vi "ReadObjectLayout.vi"(7 "properties to ignore":variant, 8 "error in (no error)":errorcluster, 10 "GObj Refnum":refnum<vi>, 11 "Control Layout in":refnum<class "Control Layout.lvclass">) -> (0 "error out":errorcluster, 3 "Control Layout out":refnum<class "Control Layout.lvclass">)   [LabVIEW 2010, in "NI_SE_Front Panel Layout.lvlib" / "Control Layout.lvclass"]
doc: "Read layout information from the GObj Refnum."
uses:
  Control Layout.lvclass
  Object Layout/Object Layout.lvclass
  Control Layout.lvclass/Control Layout.ctl
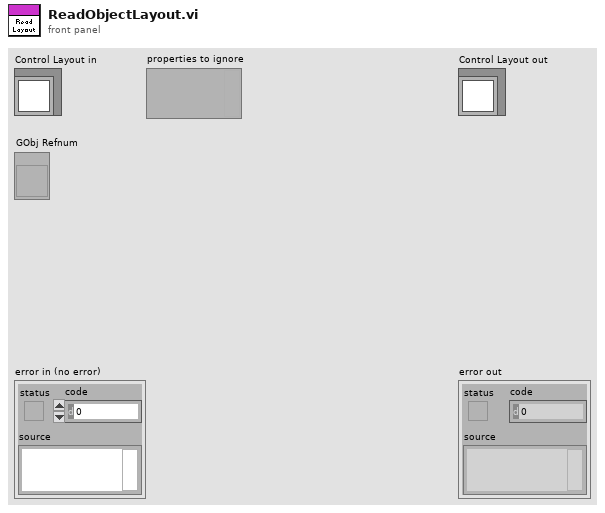
[diagram p1: front panel]
types:
  T1 = typedef "LVFontTypeDef.ctl" = cluster{"Font Name":string, "Size":u16, "Bold":bool, "Italic":bool, "Underline":bool, "Strikeout":bool, "Color":u32}
  T2 = typedef "LVPositionTypeDef.ctl" = cluster{"Left":i32, "Top":i32}
  T3 = typedef "LVBoundsTypeDef.ctl" = cluster{"Width":u32, "Height":u32}
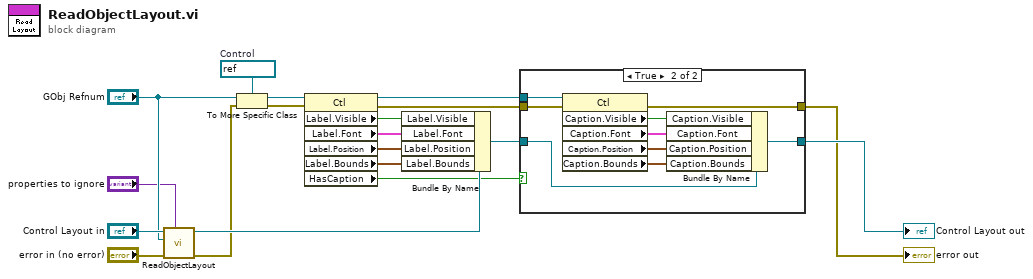
[diagram p0: block diagram]
diagram:
  w11 = refnum<vi> refnum  # Control
  n1 = call-parent "ReadObjectLayout.vi"("properties to ignore"="properties to ignore", "error in (no error)"="error in (no error)", "GObj Refnum"="GObj Refnum", "Object Layout in"="Control Layout in") -> ("error out"=w16:errorcluster, "Object Layout out"=w17:refnum<class "Control Layout.lvclass">)  [unwired: 6 in]
  n2 = To More Specific Class(target class=w11, reference="GObj Refnum", error in=w16) -> (specific class reference=w10:refnum<vi>, error out=w9:errorcluster)
  n3 = property class="Ctl"(reference=w10, error in=w9) -> (reference out=w3:refnum<vi>, error out=w4:errorcluster, "Label.Visible"=w6:bool, "Label.Font"=w7:T1, "Label.Position"=w8:T2, "Label.Bounds"=w1:T3, "HasCaption"=w5:bool)
  n4 = Bundle By Name(cluster=w17, "Label.Visible"=w6, "Label.Font"=w7, "Label.Position"=w8, "Label.Bounds"=w1) -> (w2:refnum<class "Control Layout.lvclass">)
  n5 = case shown="True" w5 {
    tunnel: w4 -> [w20 w29]
    tunnel: w3 -> [_ w30]
    tunnel: w2 -> [w21 w23]
    tunnel: [w21 w27] -> w14
    tunnel: [w20 w28] -> w13
    frame False {
    }
    frame True {
      n6 = property class="Ctl"(reference=w30, error in=w29) -> (error out=w28:errorcluster, "Caption.Visible"=w26:bool, "Caption.Font"=w25:T1, "Caption.Position"=w24:T2, "Caption.Bounds"=w22:T3)  [unwired: 1 out]
      n7 = Bundle By Name(cluster=w23, "Caption.Visible"=w26, "Caption.Font"=w25, "Caption.Position"=w24, "Caption.Bounds"=w22) -> (w27:refnum<class "Control Layout.lvclass">)
    }
  }
  "error out" <- w13
  "Control Layout out" <- w14
